vi "Delete_Placeholder.vi"   [LabVIEW 2020]
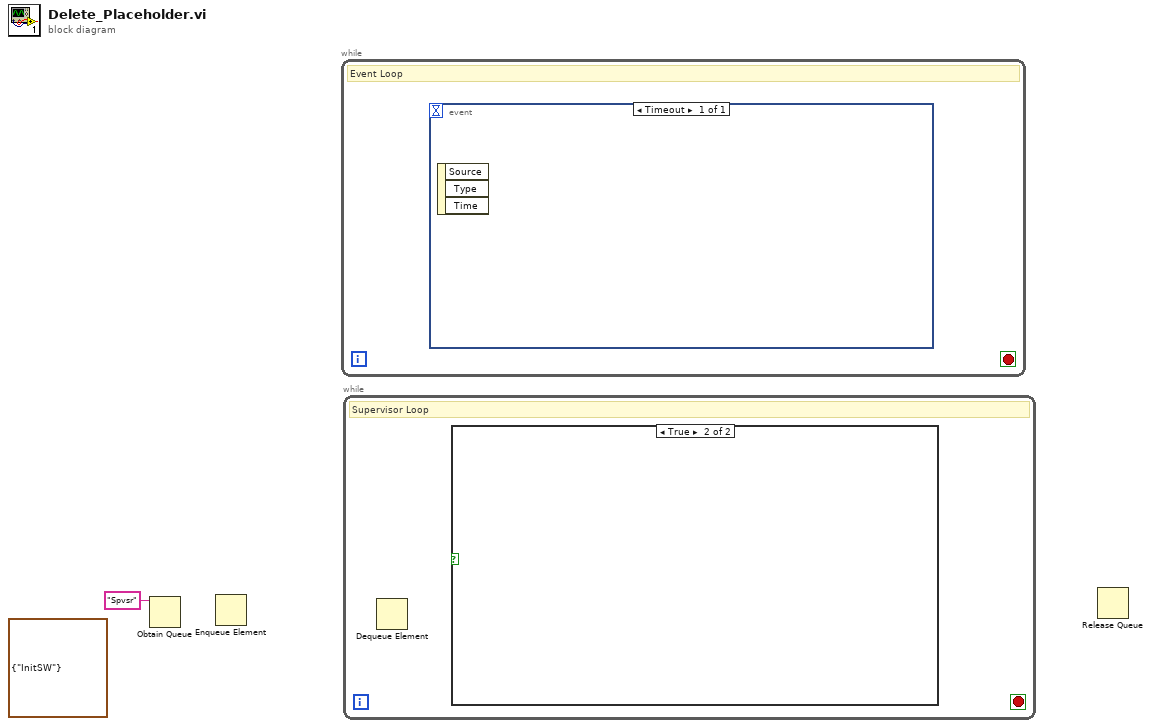
[diagram p0: block diagram]
diagram:
  (unwired) cluster{enum16{"InitSW"}} {enum."InitSW"}
  n1 = Obtain Queue(name (unnamed)="Spvsr") -> ()  [unwired: 4 in, 3 out]
  n2 = Enqueue Element() -> ()  [unwired: 4 in, 3 out]
  n3 = while {
    stop <- _ stop-if-true
    # "Event Loop"
    n4 = event shown="[0] Timeout" {
      selector: _ -> [_]
      dyn-events: _ -> [_]
      timeout: _ -> [_]
      event Timeout {
        n5 = event-data() -> ()  [unwired: 1 in, 3 out]
      }
    }
  }
  n6 = while {
    stop <- _ stop-if-true
    # "Supervisor Loop"
    n7 = Dequeue Element() -> ()  [unwired: 3 in, 4 out]
    n8 = case shown="True" {
      selector: _ -> [_ _]
      frame False {
      }
      frame True {
      }
    }
  }
  n9 = Release Queue() -> ()  [unwired: 3 in, 3 out]
